vi "VirtualBench_Acquire_Channel.vi"(11 "Acquisition Time (s)":dbl=5.0 caption="Acquisition Time (s) (no change)") -> (3 "Waveform Graph":waveform(dbl)[](graph))   [LabVIEW 2016]
uses:
  <vilib>/VirtualBench/_MSO Configure Analog Channel0.vi
  <vilib>/VirtualBench/_MSO Configure Timing12.vi
  <vilib>/VirtualBench/VirtualBench.lvlib
panel:
  in  "Vertical Offset":dbl caption="Vertical Offset (no change)"
  in  "Vertical Range":dbl=15.0 caption="Vertical Range (no change)"
  in  "Probe Attenuation":i32(ring)=1 caption="Probe Attenuation (no change)" items=["1x"=1, "10x"=10]
  in  "Sample Rate":dbl=100000.0 caption="Sample Rate (no change)"
  in  "Vertical Coupling":i32(ring)=1 caption="Vertical Coupling (no change)" items=["AC", "DC"]
  in  "Channel":tag="mso/1"
  in  "Device Name":tag="VirtualBench"
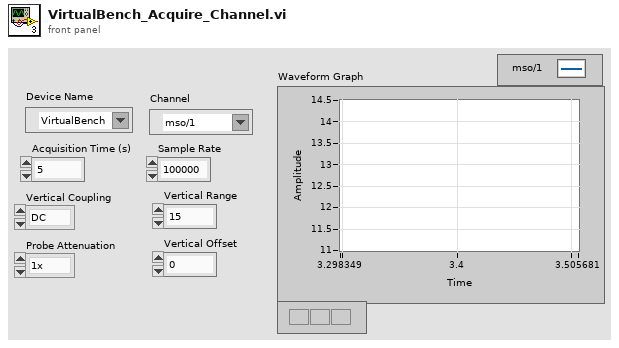
[diagram p1: front panel]
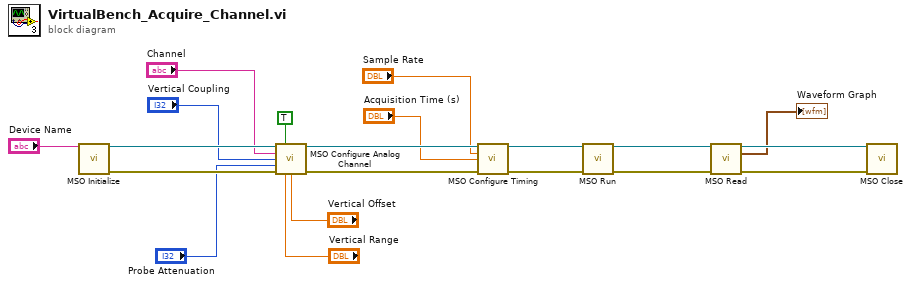
[diagram p0: block diagram]
diagram:
  n1 = call <vilib>:"MSO Initialize.vi"("Device Name"="Device Name") -> ("Instrument Handle Out"=w20:refnum<k21>, "Error Out"=w19:errorcluster)  [unwired: 13 in]
  n2 = call-poly <vilib>:"MSO Configure Analog Channel.vi"("Instrument Handle In"=w20, "Enable Channel"=TRUE, "Channel"="Channel", "Vertical Coupling"="Vertical Coupling", "Probe Attenuation"="Probe Attenuation", "Error In"=w19, "Vertical Range"="Vertical Range", "Vertical Offset"="Vertical Offset") -> ("Instrument Handle Out"=w18:refnum<k21>, "Error Out"=w17:errorcluster)  [unwired: 6 in]
  n3 = call-poly <vilib>:"MSO Configure Timing.vi"("Instrument Handle In"=w18, "Sample Rate"="Sample Rate", "Acquisition Time (s)"="Acquisition Time (s)", "Error In"=w17) -> ("Instrument Handle Out"=w16:refnum<k21>, "Error Out"=w15:errorcluster)  [unwired: 10 in]
  n4 = call <vilib>:"MSO Run.vi"("Instrument Handle In"=w16, "Error In"=w15) -> ("Instrument Handle Out"=w14:refnum<k21>, "Error Out"=w13:errorcluster)  [unwired: 12 in]
  n5 = call <vilib>:"MSO Read.vi"("Instrument Handle In"=w14, "Error In"=w13) -> ("Instrument Handle Out"=w12:refnum<k21>, "Analog Waveforms"=→"Waveform Graph":waveform(dbl)[], "Error Out"=w11:errorcluster)  [unwired: 8 in, 3 out]
  n6 = call <vilib>:"MSO Close.vi"("Instrument Handle In"=w12, "Error In"=w11) -> ()  [unwired: 13 in, 1 out]
